vi "Set Waveform AI Channel.vi"(8 "error in (no error)":errorcluster, 10 "AI Channel":i32, 11 "Waveform in":waveform(dbl)) -> (0 "error out":errorcluster, 3 "Waveform out":waveform(dbl))   [LabVIEW 2019, in "Waveform.Attributes.lvlib"]
uses:
  Waveform.Attributes.lvlib
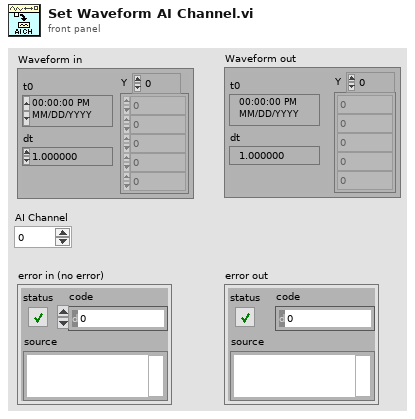
[diagram p1: front panel]
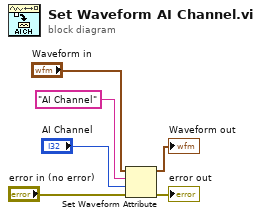
[diagram p0: block diagram]
diagram:
  n1 = Set Waveform Attribute(4:"error in (no error)", 5:"AI Channel", 6:"AI Channel" ("name"), 7:"Waveform in") -> (0:→"error out":errorcluster, 3:→"Waveform out":waveform(dbl))  [unwired: 1 out]
